vi "isNumerics.vi"(10 "Allow Complex?":bool, 11 "Type Enum":T1) -> (3 "is Numeric":bool)   [LabVIEW 2013, in "Caraya.lvlib" / "Assert.lvclass"]
uses:
  Assert.lvclass
  <vilib>/Utility/VariantDataType/Type.ctl
  <vilib>/Utility/VariantDataType/VariantType.lvlib
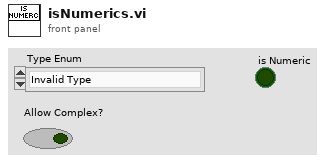
[diagram p1: front panel]
types:
  T1 = typedef "VariantType.lvlib/Type.ctl" = enum8{"Invalid Type", "Void", "I8", "I16", "I32", "I64", "U8", "U16", "U32", "U64", "Single Float", "Double Float", "Extended Float", "Single Complex", "Double Complex", "Extended Complex", "Enum U8", "Enum U16", "Enum U32", "Enum U64", "Single Float With Unit", "Double Float With Unit", "Extended Float With Unit", "Single Complex with Unit", "Double Complex with Unit", "Extended Complex with Unit", "Boolean", "String", "Path", "Picture", "Tag", "Array", "Cluster", "Variant", "LV Variant", "Waveform", "Timestamp", "Digital Waveform", "Digital Data", "ExpressData", "Refnum", "External Data", "VI", "Poly VI", "LabVIEW Class Instance", "Fixed Point"}
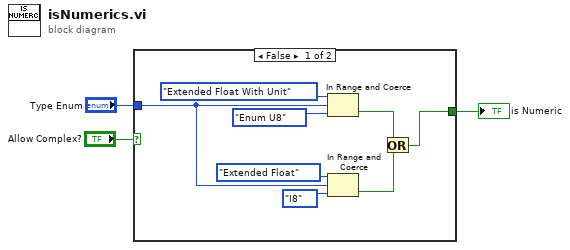
[diagram p0: block diagram]
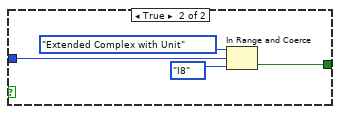
[diagram p2: hidden frame]
diagram:
  n1 = case shown="False" "Allow Complex?" {
    tunnel: "Type Enum" -> [w11 w15]
    tunnel: [w10 w12] -> w2
    frame False {
      n2 = In Range and Coerce(upper limit=Type."Extended Float With Unit" ("Type Enum"), x=w11, lower limit=Type."Enum U8" ("Type Enum")) -> (In Range?=w6:bool)  [unwired: 1 out]
      n3 = In Range and Coerce(upper limit=Type."Extended Float" ("Type Enum"), x=w11, lower limit=Type."I8" ("Type Enum")) -> (In Range?=w7:bool)  [unwired: 1 out]
      n4 = Or(x=w6, y=w7) -> (x .or. y?=w10:bool)
    }
    frame True {
      n5 = In Range and Coerce(upper limit=Type."Extended Complex with Unit" ("Type Enum"), x=w15, lower limit=Type."I8" ("Type Enum")) -> (In Range?=w12:bool)  [unwired: 1 out]
    }
  }
  "is Numeric" <- w2
